vi "DDS Generate RAM Data.vi"(8 "error in (no error)":errorcluster, 11 "DDS Channel":T3={"Power"=FALSE, "Channel Parameters"={"Ref Clock Rate [MHz]"=1000.0, "Full Scale Output\nPower [dBm]"=0.0}, "RAM Enable"=FALSE, "RAM Dest Type"=enum."Frequency", "RAM Default"={"Frequency [MHz]"=0.0, "Amplitude [dBm]"=0.0, "Phase Offset [rad]"=0.0}, "Array of DDS Profiles (8)"=[], "Description"=""} {"Array of DDS Profiles (8)"."Time Step (us)" min=0.0 max=262.14 step=0.004 format="%8.3g"; "Channel Parameters"."Ref Clock Rate [MHz]" min=0.0}) -> (0 "error out":errorcluster, 2 "RAM Profile Array":T1[](array[typedef]), 3 "RAM Word Array":u32[](array[numeric]))   [LabVIEW 2014, in "DDS.lvlib"]
uses:
  DDS.lvlib
  Controls/DDS Channel.ctl
  Controls/DDS Channel Parameters.ctl
  Controls/DDS RAM Destination.ctl
  Controls/DDS Profile Array.ctl
  Controls/DDS Profile.ctl
  Controls/DDS RAM Mode.ctl
  Controls/DDS RAM Timestep.ctl
  Controls/DDS RAM Profile.ctl
  <vilib>/gmath/NI_Gmath.lvlib
panel:
  out "Calculated Ramp":dbl[](array[numeric])
  # "f/f/A"
  # "Mag"
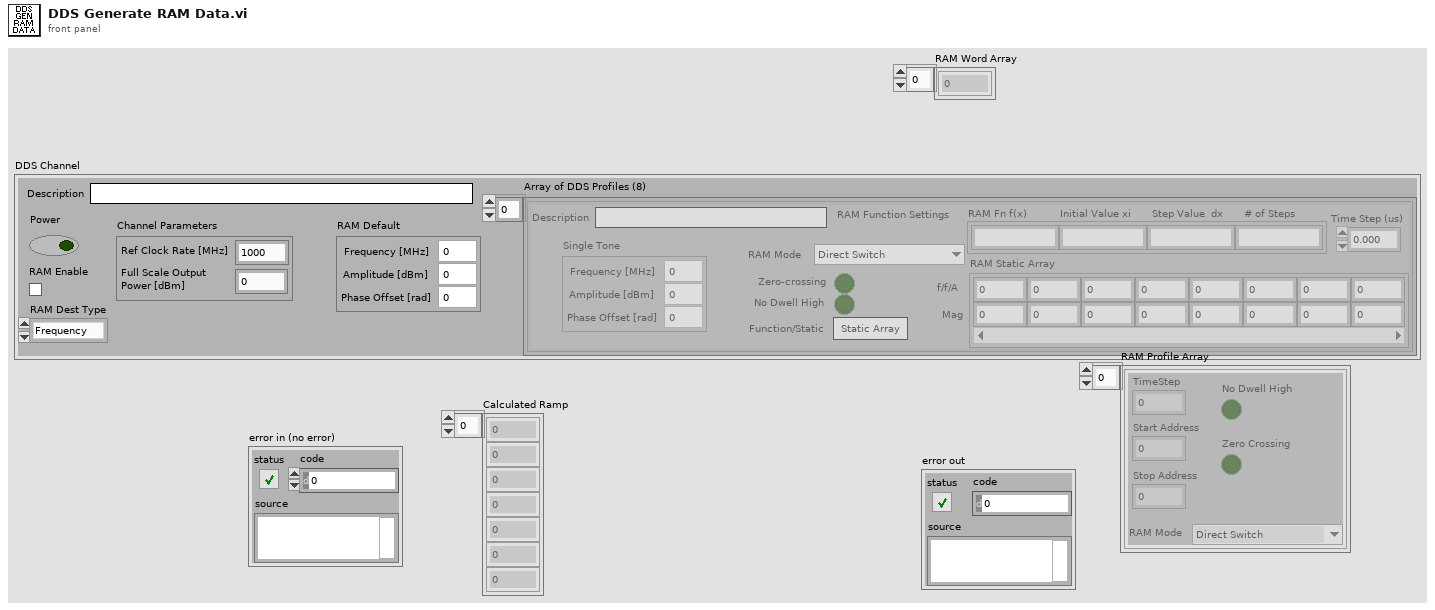
[diagram p1: front panel]
types:
  T1 = typedef "DDS.lvlib/DDS RAM Profile.ctl" = cluster{"TimeStep":u16, "Start Address":u16, "Stop Address":u16, "RAM Mode":T2, "No Dwell High":bool, "Zero Crossing":bool}
  T2 = typedef "DDS.lvlib/DDS RAM Mode.ctl" = enum16{"Direct Switch", "Ramp Up", "Bidirectional Ramp", "Continuous Bidirectional Ramp", "Continuous Recirculate", "Direct Switch 2", "Direct Switch 3", "Direct Switch 4"}
  T3 = typedef "DDS.lvlib/DDS Channel.ctl" = cluster{"Power":bool, "Channel Parameters":T4, "RAM Enable":bool, "RAM Dest Type":T5, "RAM Default":cluster{"Frequency [MHz]":dbl, "Amplitude [dBm]":dbl, "Phase Offset [rad]":dbl}, "Array of DDS Profiles (8)":T6, "Description":string}
  T4 = typedef "DDS.lvlib/DDS Channel Parameters.ctl" = cluster{"Ref Clock Rate [MHz]":dbl, "Full Scale Output\nPower [dBm]":dbl}
  T5 = typedef "DDS.lvlib/DDS RAM Destination.ctl" = enum16{"Frequency", "Phase", "Amplitude", "Polar"}
  T6 = typedef "DDS.lvlib/DDS Profile Array.ctl" = T7[]
  T7 = typedef "DDS.lvlib/DDS Profile.ctl" = cluster{"Single Tone":cluster{"Frequency [MHz]":dbl, "Amplitude [dBm]":dbl, "Phase Offset [rad]":dbl}, "RAM Mode ":T8, "Zero-crossing":bool, "No Dwell High":bool, "Function/Static":bool, "RAM Function Settings":string[], "RAM Static Array":dbl[][], "Description":string, "Time Step (us)":T9}
  T8 = typedef "DDS.lvlib/DDS RAM mode.ctl" = enum16{"Direct Switch", "Ramp Up", "Bidirectional Ramp", "Continuous Bidirectional Ramp", "Continuous Recirculate", "Direct Switch 2", "Direct Switch 3", "Direct Switch 4"}
  T9 = typedef "DDS.lvlib/DDS RAM Timestep.ctl" = dbl
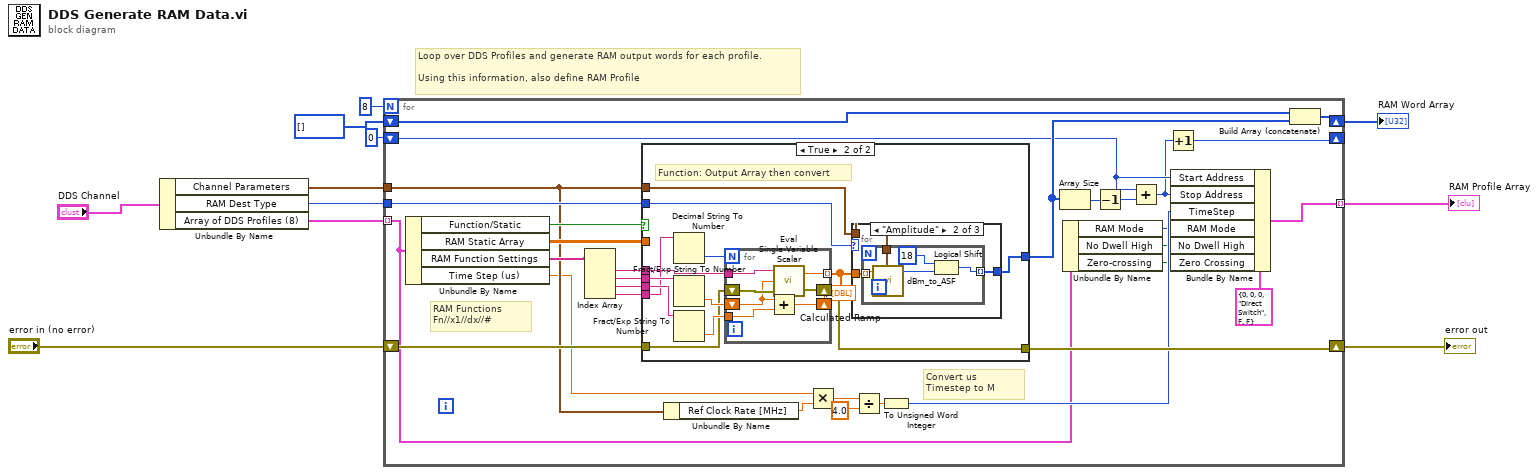
[diagram p0: block diagram]
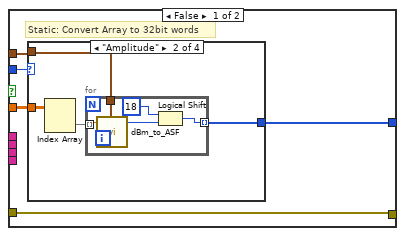
[diagram p2: hidden frame]
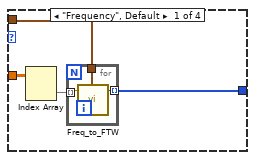
[diagram p3: hidden frame]
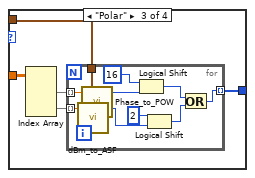
[diagram p4: hidden frame]
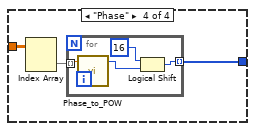
[diagram p5: hidden frame]
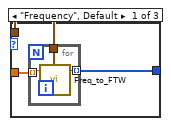
[diagram p6: hidden frame]
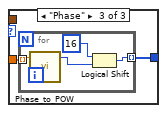
[diagram p7: hidden frame]
diagram:
  # "Loop over DDS Profiles and generate RAM output words for each profile.\n\nUsing this information, also define RAM Profile"
  n1 = Unbundle By Name("DDS Channel") -> ("Channel Parameters"=w7:T4, "RAM Dest Type"=w8:T5, "Array of DDS Profiles (8)"=w9:T6)
  n2 = for {
    N: 8 -> [_]
    tunnel: w9 -> [w14] mode=indexing
    tunnel: w8 -> [w41]
    tunnel: w7 -> [w29]
    shift-right: [w39] -> w2
    shift-left: u32[] [] -> [w38]
    shift-right: [w32] -> w3
    shift-left: "error in (no error)" -> [w33]
    tunnel: [w25] -> w1 mode=indexing
    shift-right: [w19] -> _
    shift-left: u16 0 -> [w21]
    # "Convert us Timestep to M"
    # "RAM Functions\nFn//x1//dx//#"
    n3 = Unbundle By Name(w14) -> ("Function/Static"=w42:bool, "RAM Static Array"=w40:dbl[][], "RAM Function Settings"=w37:string[], "Time Step (us)"=w12:T9)
    n4 = Index Array(array=w37) -> (element #1=w36:string, element #2=w35:string, element #3=w34:string, element #4=w13:string)  [unwired: 4 in]
    n5 = case shown="True" w42 {
      tunnel: w41 -> [w47 w95]
      tunnel: w40 -> [w46 _]
      tunnel: w29 -> [w45 w94]
      tunnel: [w44 w92] -> w24
      tunnel: w36 -> [_ w91]
      tunnel: w35 -> [_ w90]
      tunnel: w34 -> [_ w89]
      tunnel: w13 -> [_ w88]
      tunnel: w33 -> [w43 w87]
      tunnel: [w43 w86] -> w32
      frame False {
        # "Static: Convert Array to 32bit words"
        n6 = case shown="\"Amplitude\"" w47 {
          tunnel: w46 -> [w51 w58 w68 w81]
          tunnel: w45 -> [w49 w56 w66 _]
          tunnel: [w48 w55 w65 w79] -> w44
          frame "Frequency", Default {
            n7 = Index Array(array=w51) -> (element=w50:dbl[])  [unwired: 2 in]
            n8 = for {
              tunnel: w50 -> [w54] mode=indexing
              tunnel: [w53] -> w48 mode=indexing
              tunnel: w49 -> [w52]
              n9 = call "Freq_to_FTW.vi"("Frequency (MHz)"=w54, "Channel Parameters"=w52) -> ("FTW (32bit)"=w53:u32)  [unwired: 25 in]
            }
          }
          frame "Amplitude" {
            n10 = Index Array(array=w58) -> (element=w57:dbl[])  [unwired: 2 in]
            n11 = for {
              tunnel: w57 -> [w63] mode=indexing
              tunnel: [w59] -> w55 mode=indexing
              tunnel: w56 -> [w62]
              n12 = call "dBm_to_ASF.vi"("Amplitude (dBm)"=w63, "Channel Parameters"=w62) -> ("ASF"=w61:u32)  [unwired: 25 in]
              n13 = Logical Shift(y=i8 18, x=w61) -> (x << y=w59:u32)
            }
          }
          frame "Polar" {
            n14 = Index Array(array=w68) -> (element #1=w67:dbl[], element #2=w64:dbl[])  [unwired: 4 in]
            n15 = for {
              tunnel: w67 -> [w73] mode=indexing
              tunnel: [w69] -> w65 mode=indexing
              tunnel: w66 -> [w78]
              tunnel: w64 -> [w76] mode=indexing
              n16 = call "dBm_to_ASF.vi"("Amplitude (dBm)"=w76, "Channel Parameters"=w78) -> ("ASF"=w75:u32)  [unwired: 25 in]
              n17 = call "Phase_to_POW.vi"("Phase (rad.)"=w73) -> ("POW"=w72:u32)  [unwired: 26 in]
              n18 = Logical Shift(y=i8 16, x=w72) -> (x << y=w70:u32)
              n19 = Logical Shift(y=i8 2, x=w75) -> (x << y=w71:u32)
              n20 = Or(x=w70, y=w71) -> (x .or. y?=w69:u32)
            }
          }
          frame "Phase" {
            n21 = Index Array(array=w81) -> (element=w80:dbl[])  [unwired: 2 in]
            n22 = for {
              tunnel: w80 -> [w85] mode=indexing
              tunnel: [w82] -> w79 mode=indexing
              n23 = call "Phase_to_POW.vi"("Phase (rad.)"=w85) -> ("POW"=w84:u32)  [unwired: 26 in]
              n24 = Logical Shift(y=i8 16, x=w84) -> (x << y=w82:u32)
            }
          }
        }
      }
      frame True {
        # "Function: Output Array then convert"
        n25 = Decimal String To Number(string=w88) -> (number=w96:i32)  [unwired: 2 in, 1 out]
        n26 = Fract/Exp String To Number(string=w90) -> (number=w98:dbl)  [unwired: 3 in, 1 out]
        n27 = Fract/Exp String To Number(string=w89) -> (number=w97:dbl)  [unwired: 3 in, 1 out]
        n28 = for {
          N: w96 -> [_]
          tunnel: w91 -> [w125]
          tunnel: [w124] -> w93 mode=indexing
          shift-right: [w123] -> _
          shift-left: w98 -> [w120]
          tunnel: w97 -> [w119]
          shift-right: [w122] -> w86
          shift-left: w87 -> [w121]
          n29 = Add(x=w120, y=w119) -> (x+y=w123:dbl)
          n30 = call <vilib>:"Eval Single-Variable Scalar.vi"("error in (no error)"=w121, "x value"=w120, "formula"=w125) -> ("error out"=w122:errorcluster, "y value"=w124:dbl)
        }
        "Calculated Ramp" <- w93
        n31 = case shown="\"Amplitude\"" w95 {
          tunnel: w94 -> [w101 w107 _]
          tunnel: [w100 w106 w114] -> w92
          tunnel: w93 -> [w99 w105 w113]
          frame "Frequency", Default {
            n32 = for {
              tunnel: w99 -> [w104] mode=indexing
              tunnel: [w103] -> w100 mode=indexing
              tunnel: w101 -> [w102]
              n33 = call "Freq_to_FTW.vi"("Frequency (MHz)"=w104, "Channel Parameters"=w102) -> ("FTW (32bit)"=w103:u32)  [unwired: 25 in]
            }
          }
          frame "Amplitude" {
            n34 = for {
              tunnel: w105 -> [w112] mode=indexing
              tunnel: [w108] -> w106 mode=indexing
              tunnel: w107 -> [w111]
              n35 = call "dBm_to_ASF.vi"("Amplitude (dBm)"=w112, "Channel Parameters"=w111) -> ("ASF"=w110:u32)  [unwired: 25 in]
              n36 = Logical Shift(y=i8 18, x=w110) -> (x << y=w108:u32)
            }
          }
          frame "Phase" {
            n37 = for {
              tunnel: w113 -> [w118] mode=indexing
              tunnel: [w115] -> w114 mode=indexing
              n38 = call "Phase_to_POW.vi"("Phase (rad.)"=w118) -> ("POW"=w117:u32)  [unwired: 26 in]
              n39 = Logical Shift(y=i8 16, x=w117) -> (x << y=w115:u32)
            }
          }
        }
      }
    }
    n40 = Unbundle By Name(w29) -> ("Ref Clock Rate [MHz]"=w28:dbl)
    n41 = Multiply(x=w12, y=w28) -> (x*y=w31:T9)
    n42 = Divide(x=w31, y=4.0) -> (x/y=w27:T9)
    n43 = To Unsigned Word Integer(number=w27) -> (unsigned 16bit integer=w18:u16)
    n44 = Array Size(array=w24) -> (size(s)=w23:i32)
    n45 = Unbundle By Name(w14) -> ("RAM Mode"=w17:T8, "No Dwell High"=w16:bool, "Zero-crossing"=w15:bool)
    n46 = Decrement(x=w23) -> (x-1=w22:i32)
    n47 = Add(x=w21, y=w22) -> (x+y=w20:i32)
    n48 = Increment(x=w20) -> (x+1=w19:i32)
    n49 = Bundle By Name(cluster=T1 {"TimeStep"=0, "Start Address"=0, "Stop Address"=0, "RAM Mode"=enum."Direct Switch", "No Dwell High"=FALSE, "Zero Crossing"=FALSE} ("Cluster"), "Start Address"=w21, "Stop Address"=w20, "TimeStep"=w18, "RAM Mode"=w17, "No Dwell High"=w16, "Zero Crossing"=w15) -> (w25:T1)
    n50 = Build Array (concatenate)(w38, w24) -> (w39:u32[])
  }
  "error out" <- w3
  "RAM Word Array" <- w2
  "RAM Profile Array" <- w1
